vi "add channel to configuration.vi"(8 "error in":errorcluster, 10 "channel":refnum<class "TBM channel.lvclass">, 11 "UI Reference configuration in":refnum<class "UI Reference configuration.lvclass">) -> (0 "error out":errorcluster, 3 "UI Reference configuration out":refnum<class "UI Reference configuration.lvclass">)   [LabVIEW 2013, in "UI Reference configuration.lvclass"]
uses:
  UI Reference configuration.lvclass
  <vilib>/NI/Tag Bus Module Framework/channel/TBM channel.lvclass
  <vilib>/NI/Tag Bus/tag/tag descriptor.lvclass/tag descriptor.ctl
  UI Reference configuration.lvclass/UI Reference configuration.ctl
  <vilib>/NI/Tag Bus/tag/tag descriptor.lvclass
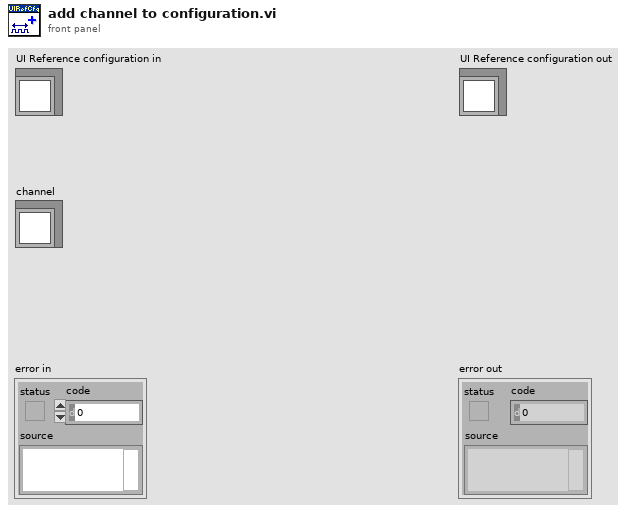
[diagram p1: front panel]
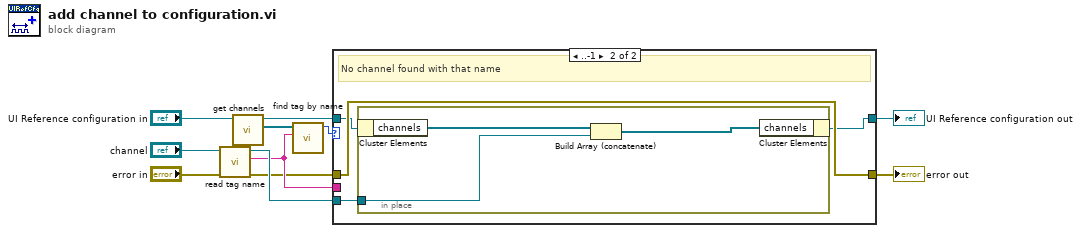
[diagram p0: block diagram]
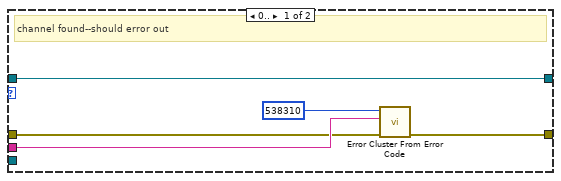
[diagram p2: hidden frame]
diagram:
  n1 = call <vilib>:"read tag name.vi"("error in"="error in", "system tag in"="channel") -> ("error out"=w2:errorcluster, "name"=w3:string, "system tag out"=w10:refnum<class "TBM channel.lvclass">)  [unwired: 7 in]
  n2 = call-dynamic "get channels.vi"("UI Reference configuration in"="UI Reference configuration in") -> ("channels"=w5:refnum<class "TBM channel.lvclass">[], "UI Reference configuration out"=w11:refnum<class "UI Reference configuration.lvclass">)  [unwired: 9 in]
  n3 = call <vilib>:"find tag by name.vi"("name"=w3, "tags in"=w5) -> ("index"=w4:i32)  [unwired: 9 in]
  n4 = case shown="..-1" w4 {
    tunnel: [w16 w19] -> w8
    tunnel: w3 -> [w14 _]
    tunnel: w2 -> [w13 w19]
    tunnel: w11 -> [w12 w18]
    tunnel: w10 -> [_ w20]
    tunnel: [w12 w17] -> w7
    frame 0.. {
      # "channel found--should error out"
      n5 = call <vilib>:"Error Cluster From Error Code.vi"("error in (no error)"=w13, "error message (\"\")"=w14, "error code (0)"=538310) -> ("error out"=w16:errorcluster)  [unwired: 6 in]
    }
    frame ..-1 {
      # "No channel found with that name"
      n6 = in-place {
        in-place-border: w20 -> [w23]
        n7 = in-place-cluster #1(w18) -> ("channels"=w21:refnum<class "TBM channel.lvclass">[])
        n8 = Build Array (concatenate)(w21, w23) -> (w22:refnum<class "TBM channel.lvclass">[])
        n9 = in-place-cluster #1("channels"=w22) -> (w17:refnum<class "UI Reference configuration.lvclass">)
      }
    }
  }
  "error out" <- w8
  "UI Reference configuration out" <- w7
